vi "Switch Fail Warning.vi"(11 "Switch Unit":T1=enum."Pickering") -> (0 "Retry":bool, 3 "Switch Unit":T1=enum."Pickering")   [LabVIEW 2022 SP3]
uses:
  SwitchOption.ctl
  SwitchGlobals.vi
panel:
  in  "USB Switch":string
  out "User Message":string
  in  "Abort":bool
  in  "Try Again":bool
  # "Switch Initialization Failed!"
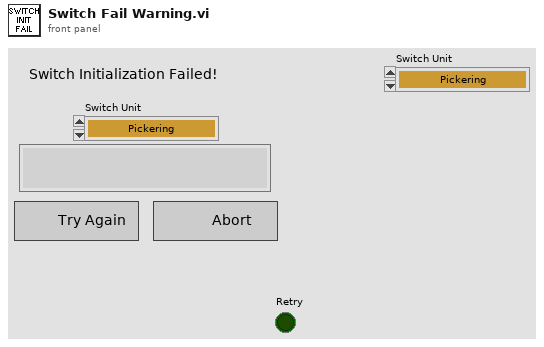
[diagram p1: front panel]
types:
  T1 = typedef "SwitchOption.ctl" = enum16{"Cytex", "Pickering", "NI Switch", "No Switch", "Riverside USB"}
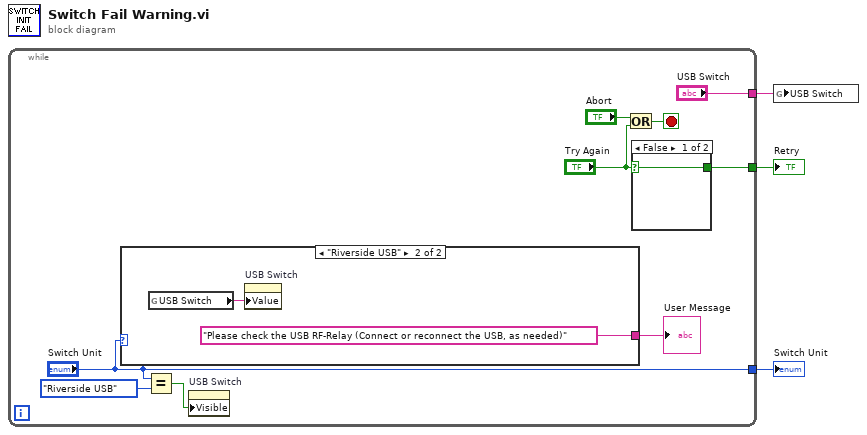
[diagram p0: block diagram]
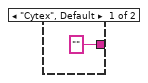
[diagram p2: hidden frame]
diagram:
  n1 = while {
    tunnel: ["Switch Unit"] -> w2
    tunnel: [w9] -> w3
    tunnel: ["USB Switch"] -> w1
    stop <- w11 stop-if-true
    n2 = case shown="\"Riverside USB\"" "Switch Unit" {
      tunnel: ["" "Please check the USB RF-Relay (Connect or reconnect the USB, as needed)"] -> w8
      frame "Cytex", Default {
      }
      frame "Riverside USB" {
        n3 = global read "SwitchGlobals.vi" "USB Switch"() -> (w14:string)
        n4 = property on="USB Switch" class="Str"("Value"=w14) -> ()  [unwired: 2 in, 2 out]
      }
    }
    "User Message" <- w8
    n5 = Equal?(x="Switch Unit", y=SwitchOption."Riverside USB") -> (x = y?=w4:bool)
    n6 = property on="USB Switch" class="Str"("Visible"=w4) -> ()  [unwired: 2 in, 2 out]
    n7 = Or(x="Abort", y="Try Again") -> (x .or. y?=w11:bool)
    n8 = case shown="False" "Try Again" {
      selector: "Try Again" -> [w16 w17]
      tunnel: [w16 w17] -> w9
      frame False {
      }
      frame True {
      }
    }
  }
  "Retry" <- w3
  "Switch Unit" <- w2
  n9 = global write "SwitchGlobals.vi" "USB Switch"(w1) -> ()
